vi "Read Content.vi"(8 "Error In":errorcluster, 11 "Comment In":refnum<class "Comment.lvclass">) -> (0 "Error Out":errorcluster, 2 "Content":string, 3 "Comment Out":refnum<class "Comment.lvclass">)   [LabVIEW 2018, in "Toolkit.lvlib" / "Tokens.lvlib" / "Comment.lvclass"]
uses:
  Comment.lvclass
  Comment.lvclass/Comment.ctl
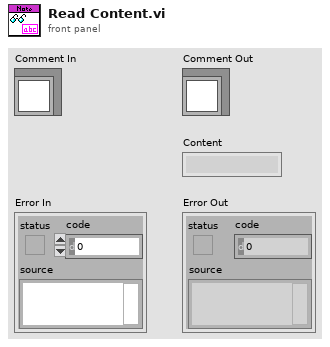
[diagram p1: front panel]
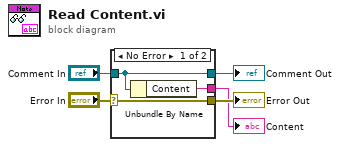
[diagram p0: block diagram]
diagram:
  n1 = case shown="No Error" "Error In" {
    selector: "Error In" -> [w8 w9]
    tunnel: [w8 w9] -> w4
    tunnel: [w7 w10] -> w2
    tunnel: "Comment In" -> [w7 w10]
    tunnel: [w6 _] -> w1
    frame No Error {
      n2 = Unbundle By Name(w7) -> ("Content"=w6:string)
    }
    frame Error {
    }
  }
  "Error Out" <- w4
  "Comment Out" <- w2
  "Content" <- w1
